vi "NIDMM_Acq Multiple Samples.vi"(0 "Device Name":refnum<k15>="Dev1", 1 "Sample Interval (sec)":dbl=1.0, 5 "Measurement Type":T1, 7 "Range":dbl=10.0 format="%.2p", 9 "Resolution (Digits)":dbl(ring)=5.5 items=["3 1/2"=3.5, "4 1/2"=4.5, "5 1/2"=5.5, "6 1/2"=6.5, "7 1/2"=7.5], 11 "error in (no error)":errorcluster, 12 "Sample Count":i32=10) -> (4 "Result":dbl, 15 "error out":errorcluster)   [LabVIEW 2015]
doc: "This example acquires multiple measurements. Select the measurement function, range, and absolute resolution. Specify the number of samples to acquire. The Read function is used to acquire the requested number of points. The data is displayed in a waveform graph.\n\nSupported Devices: 4050, 4060, 4065, 4070, 4071, 4072"
uses:
  <instrlib>/niDMM/nidmm.llb/niDMM Function.ctl
  <instrlib>/niDMM/nidmm.llb/niDMM Sample Trigger.ctl
  <instrlib>/niDMM/nidmm.llb/niDMM Configure Measurement Digits.vi
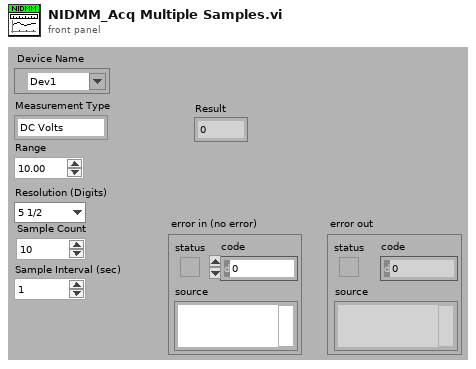
[diagram p1: front panel]
types:
  T1 = typedef "niDMM Function.ctl" = enum16{"DC Volts", "AC Volts", "DC Current", "AC Current", "2-wire Resistance", "4-wire Resistance", "Diode", "Frequency", "Period", "AC Volts DC Coupled", "Capacitance", "Inductance", "Temperature"}
  T2 = typedef "niDMM Sample Trigger.ctl" = enum16{"Immediate", "External", "TTL 0", "TTL 1", "TTL 2", "TTL 3", "TTL 4", "TTL 5", "TTL 6", "Interval", "Software", "TTL 7", "PXI Star", "LBR Trig 1", "Aux Trig 1"}
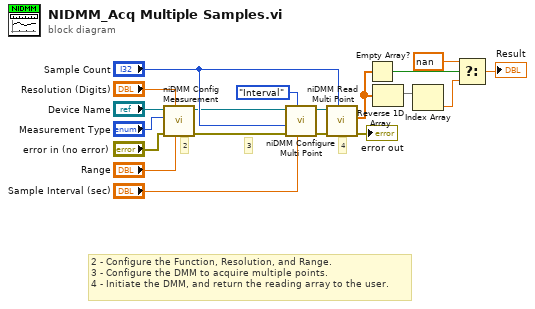
[diagram p0: block diagram]
diagram:
  # "4"
  # "2 - Configure the Function, Resolution, and Range.\n3 - Configure the DMM to acquire multiple points.\n4 - Initiate the DMM, and return the reading array to the user."
  # "3"
  # "2"
  n1 = call-poly <instrlib>:"niDMM Config Measurement.vi"("Range"="Range", "Resolution in Digits"="Resolution (Digits)", "error in (no error)"="error in (no error)", "Function"="Measurement Type", "instrument handle"="Device Name") -> ("error out"=w12:errorcluster, "instrument handle out"=w13:refnum<k15>)  [unwired: 5 in]
  n2 = call <instrlib>:"niDMM Configure Multi Point.vi"("Sample Interval (sec)"="Sample Interval (sec)", "Sample Trigger"=niDMM_Sample_Trigger."Interval", "error in (no error)"=w12, "Sample Count"="Sample Count", "instrument handle"=w13) -> ("error out"=w17:errorcluster, "instrument handle out"=w18:refnum<k15>)  [unwired: 5 in]
  n3 = call <instrlib>:"niDMM Read Multi Point.vi"("Number to Read"="Sample Count", "error in (no error)"=w17, "instrument handle"=w18) -> ("error out"=→"error out":errorcluster, "Measurements"=w5:dbl[])  [unwired: 5 in, 2 out]
  n4 = Empty Array?(array=w5) -> (empty?=w4:bool)
  n5 = Reverse 1D Array(array=w5) -> (reversed array=w6:dbl[])
  n6 = Index Array(array=w6) -> (element=w3:dbl)  [unwired: 1 in]
  n7 = Select(t=nan, s=w4, f=w3) -> (s? t:f=→"Result":dbl)
